vi "QSM - Application.vi"(8 "Error In":errorcluster) -> (0 "Error Out":errorcluster)   [LabVIEW 2023, in "QSM - IODocs.lvlib"]
doc: "This VI is the Queued State Machine for the Queued State Machine template."
uses:
  QSM - IODocs.lvlib
  Controls/State Machine Information.ctl
  Controls/State Machine Message.ctl
  Controls/Message Queue Element Position.ctl
  SubVIs/Enqueue Message (Single).vi
types:
  T1 = typedef "QSM - IODocs.lvlib/State Machine Message.ctl" = enum16{"Initialize", "Handle Error", "Exit"}
  T2 = typedef "QSM - IODocs.lvlib/State Machine Information.ctl" = cluster{"Placeholder Data":string}
  T3 = typedef "QSM - IODocs.lvlib/Message Queue Element Position.ctl" = enum16{"Front", "Back"}
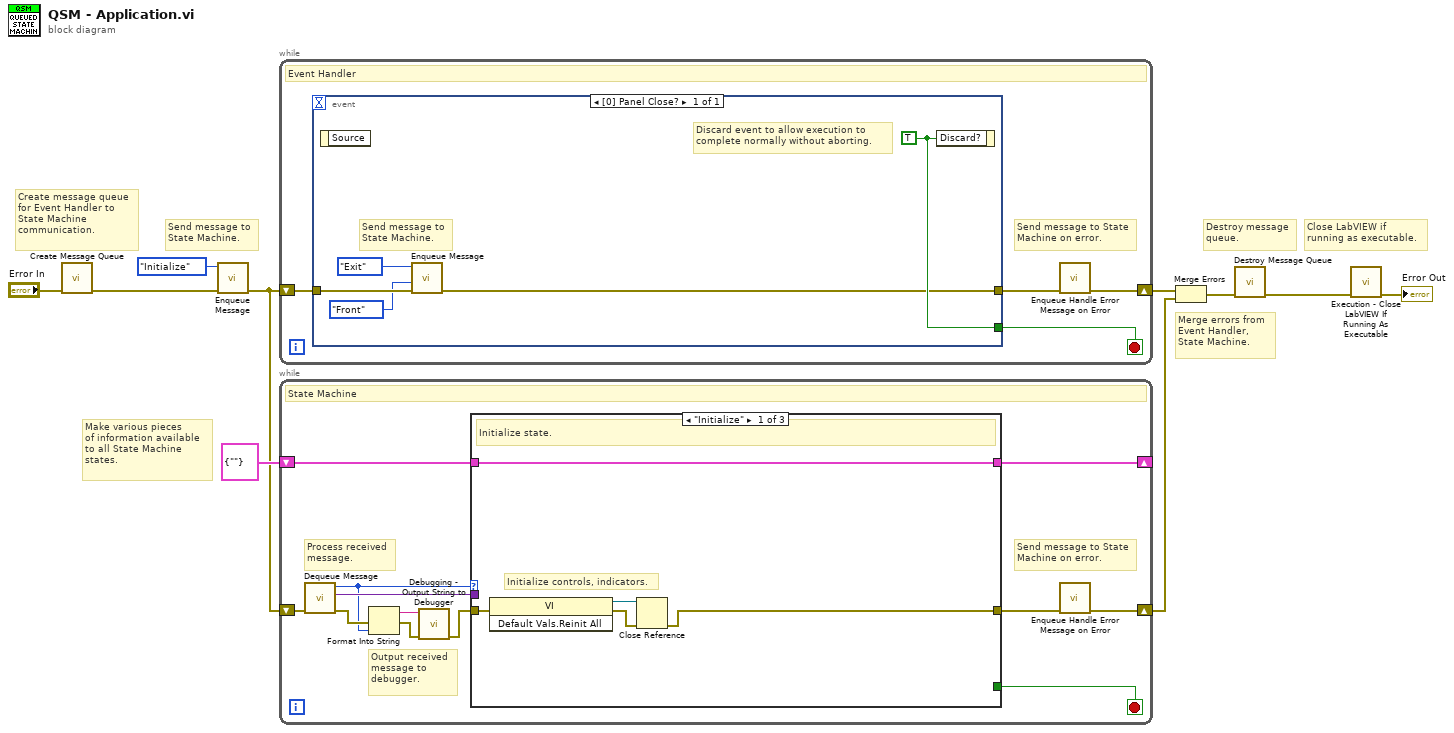
[diagram p0: block diagram]
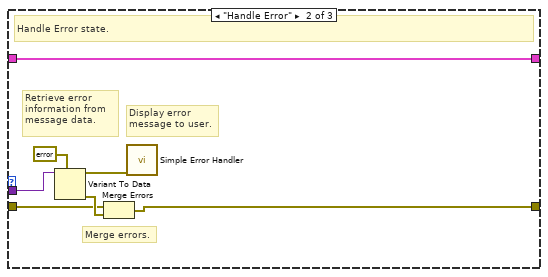
[diagram p2: hidden frame]
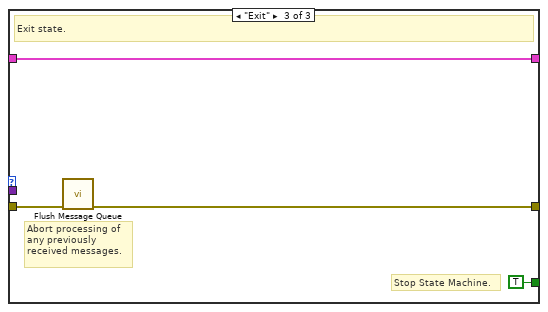
[diagram p3: hidden frame]
diagram:
  # "Close LabVIEW if\nrunning as executable."
  # "Destroy message\nqueue."
  # "Merge errors from\nEvent Handler,\nState Machine."
  # "Create message queue\nfor Event Handler to\nState Machine\ncommunication."
  # "Send message to\nState Machine."
  # "Make various pieces\nof information available\nto all State Machine\nstates."
  n1 = call "Create Message Queue.vi"("Error In"="Error In") -> ("Error Out"=w6:errorcluster)  [unwired: 10 in]
  n2 = call-poly "Enqueue Message.vi"("Error In"=w6, "State Machine Message"=State_Machine_Message."Initialize" ("State Machine State")) -> ("Error Out"=w5:errorcluster)  [unwired: 9 in]
  n3 = while {
    shift-right: [w12] -> w10
    shift-left: w5 -> [w14]
    stop <- w11 stop-if-true
    # "Send message to State\nMachine on error."
    # "Event Handler"
    n4 = event shown="[0] Panel Close?" {
      selector: _ -> [_]
      dyn-events: _ -> [_]
      timeout: _ -> [_]
      tunnel: [w19] -> w11
      tunnel: w14 -> [w18]
      tunnel: [w17] -> w13
      event Panel Close? {
        w19 = TRUE ("Discard?")
        # "Send message to\nState Machine."
        # "Discard event to allow execution to\ncomplete normally without aborting."
        n5 = event-data() -> ()  [unwired: 1 in, 1 out]
        n6 = call-poly "Enqueue Message.vi"("Error In"=w18, "Message Position"=Message_Queue_Element_Position."Front", "State Machine Message"=State_Machine_Message."Exit" ("State Machine State")) -> ("Error Out"=w17:errorcluster)  [unwired: 8 in]
        n7 = event-data("Discard?"=w19) -> ()  [unwired: 1 in, 1 out]
      }
    }
    n8 = call "Enqueue Handle Error Message on Error.vi"("Error In"=w13) -> ("Error Out"=w12:errorcluster)  [unwired: 10 in]
  }
  n9 = while {
    shift-right: [w22] -> w9
    shift-left: w5 -> [w29]
    shift-right: [w30] -> _
    shift-left: T2 {"Placeholder Data"=""} ("State Machine Information") -> [w31]
    stop <- w20 stop-if-true
    # "Send message to State\nMachine on error."
    # "Output received\nmessage to\ndebugger."
    # "Process received\nmessage."
    # "State Machine"
    n10 = call "Dequeue Message.vi"("Error In"=w29) -> ("Error Out"=w26:errorcluster, "Data"=w28:variant, "State Machine Message"=w24:T1)  [unwired: 8 in]
    n11 = Format Into String(error in=w26, w24) -> (resulting string=w21:string, error out=w27:errorcluster)  [unwired: 2 in]
    n12 = call "Debugging - Output String to Debugger.vi"("Error In"=w27, "String"=w21) -> ("Error Out"=w25:errorcluster)  [unwired: 9 in]
    n13 = case shown="\"Initialize\"" w24 {
      tunnel: w25 -> [w33 w38 w44]
      tunnel: [w34 w39 w45] -> w23
      tunnel: [_ _ TRUE ("Discard?")] -> w20
      tunnel: w31 -> [w32 w43 w46]
      tunnel: [w32 w43 w46] -> w30
      tunnel: w28 -> [_ w37 _]
      frame "Initialize" {
        # "Initialize controls, indicators."
        # "Initialize state."
        n14 = invoke class="VI" method="Default Vals.Reinit All"(error in=w33) -> (reference out=w36:refnum<vi>, error out=w35:errorcluster)  [unwired: 2 in, 1 out]
        n15 = Close Reference(reference=w36, error in (no error)=w35) -> (error out=w34:errorcluster)
      }
      frame "Handle Error" {
        # "Merge errors."
        # "Retrieve error\ninformation from\nmessage data."
        # "Display error\nmessage to user."
        # "Handle Error state."
        n16 = Variant To Data(type=errorcluster {"status"=FALSE, "code"=0, "source"=""} ("error in (no error)"), Variant=w37) -> (data=w41:errorcluster, error out=w42:errorcluster)  [unwired: 1 in]
        n17 = Merge Errors(w38, w42) -> (w39:errorcluster)
        n18 = call <vilib>:"Simple Error Handler.vi"("error in (no error)"=w41) -> ()  [unwired: 4 in, 5 out]
      }
      frame "Exit" {
        # "Stop State Machine."
        # "Abort processing of\nany previously\nreceived messages."
        # "Exit state."
        n19 = call "Flush Message Queue.vi"("Error In"=w44) -> ("Error Out"=w45:errorcluster)  [unwired: 9 in, 1 out]
      }
    }
    n20 = call "Enqueue Handle Error Message on Error.vi"("Error In"=w23) -> ("Error Out"=w22:errorcluster)  [unwired: 10 in]
  }
  n21 = Merge Errors(w10, w9) -> (w4:errorcluster)
  n22 = call "Destroy Message Queue.vi"("Error In"=w4) -> ("Error Out"=w2:errorcluster)  [unwired: 10 in]
  n23 = call "Execution - Close LabVIEW If Running As Executable.vi"("Error In"=w2) -> ("Error Out"=→"Error Out":errorcluster)  [unwired: 10 in]
